vi "LVUT_MainSequence(Example).vi"(8 "error in (no error)":errorcluster) -> (0 "error out":errorcluster)   [LabVIEW 2019, in "Sequence Example.lvlib"]
uses:
  Sequence Example.lvlib
  Unit Test Engine Tools.lvlib
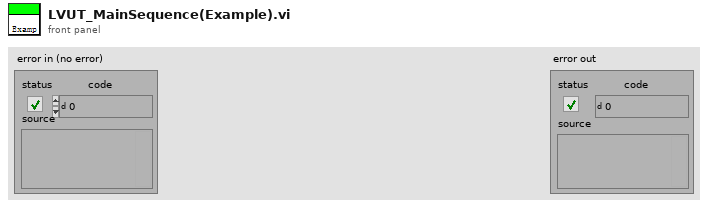
[diagram p1: front panel]
types:
  T1 = enum16{"Station 1", "Station 2", "Station 3", "Station 4"}
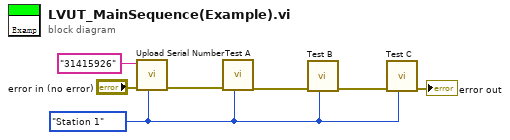
[diagram p0: block diagram]
diagram:
  w3 = T1."Station 1" ("Station")
  n1 = call "Upload Serial Number.vi"("Station"=w3, "error in (no error)"="error in (no error)", "SerialNumber"="31415926") -> ("error out"=w5:errorcluster)  [unwired: 8 in]
  n2 = call "Test A.vi"("Station"=w3, "error in (no error)"=w5) -> ("error out"=w7:errorcluster)  [unwired: 9 in]
  n3 = call "Test B.vi"("Station"=w3, "error in (no error)"=w7) -> ("error out"=w6:errorcluster)  [unwired: 9 in]
  n4 = call "Test C.vi"("Station"=w3, "error in (no error)"=w6) -> ("error out"=→"error out":errorcluster)  [unwired: 9 in]
